vi "Timer.vi"(9 "Delay (sec)":dbl=10.0, 11 "Reset timer":bool) -> (0 "End Time":string, 1 "Current Time":string, 2 "Start Time":string, 3 "Time Elapsed":bool)   [LabVIEW 2022 SP3]
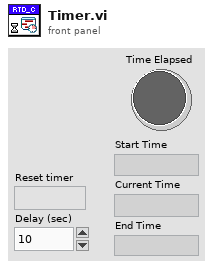
[diagram p1: front panel]
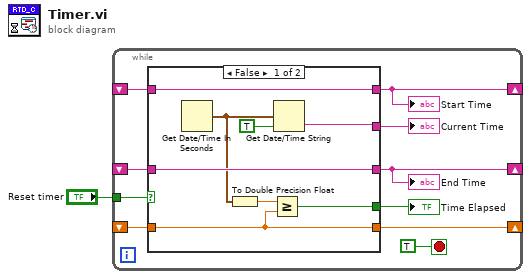
[diagram p0: block diagram]
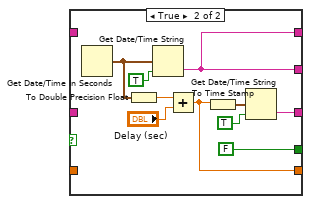
[diagram p2: hidden frame]
diagram:
  n1 = while {
    tunnel: "Reset timer" -> [w10]
    shift-right: [w6] -> _
    shift-left: _ -> [w8]
    shift-right: [w4] -> _
    shift-left: _ -> [w5]
    shift-right: [w3] -> _
    shift-left: _ -> [w2]
    stop <- TRUE stop-if-true
    n2 = case shown="False" w10 {
      tunnel: [w18 w21] -> w9
      tunnel: [w16 w24] -> w6
      tunnel: w8 -> [w16 _]
      tunnel: [w17 FALSE] -> w7
      tunnel: [w15 w21] -> w4
      tunnel: w5 -> [w15 _]
      tunnel: [w14 w20] -> w3
      tunnel: w2 -> [w14 _]
      frame False {
        n3 = Get Date/Time In Seconds() -> (seconds since 1Jan1904=w13:timestamp)
        n4 = To Double Precision Float(number=w13) -> (double precision float=w12:dbl)
        n5 = Greater Or Equal?(x=w12, y=w14) -> (x >= y?=w17:bool)
        n6 = Get Date/Time String(seconds (now)=w13, want seconds? (F)=TRUE) -> (time string=w18:string)  [unwired: 1 in, 1 out]
      }
      frame True {
        n7 = Get Date/Time In Seconds() -> (seconds since 1Jan1904=w27:timestamp)
        n8 = To Double Precision Float(number=w27) -> (double precision float=w29:dbl)
        n9 = Get Date/Time String(seconds (now)=w27, want seconds? (F)=TRUE) -> (time string=w21:string)  [unwired: 1 in, 1 out]
        n10 = Add(x=w29, y="Delay (sec)") -> (x+y=w20:dbl)
        n11 = To Time Stamp(1:w20) -> (0:w28:timestamp)
        n12 = Get Date/Time String(seconds (now)=w28, want seconds? (F)=TRUE) -> (time string=w24:string)  [unwired: 1 in, 1 out]
      }
    }
    "Current Time" <- w9
    "Time Elapsed" <- w7
    "End Time" <- w6
    "Start Time" <- w4
  }
